vi "Write Default channels.vi"(8 "error in (no error)":errorcluster, 9 "Keep old\nplots":bool, 10 "Default channels":string[][](array[string]), 11 "Common Measurements in":refnum<class "Common Measurements.lvclass">) -> (0 "error out":errorcluster, 3 "Common Measurements out":refnum<class "Common Measurements.lvclass">)   [LabVIEW 2015, in "Common Measurements.lvclass"]
uses:
  Common Measurements.lvclass
  Common Measurements.lvclass/Common Measurements.ctl
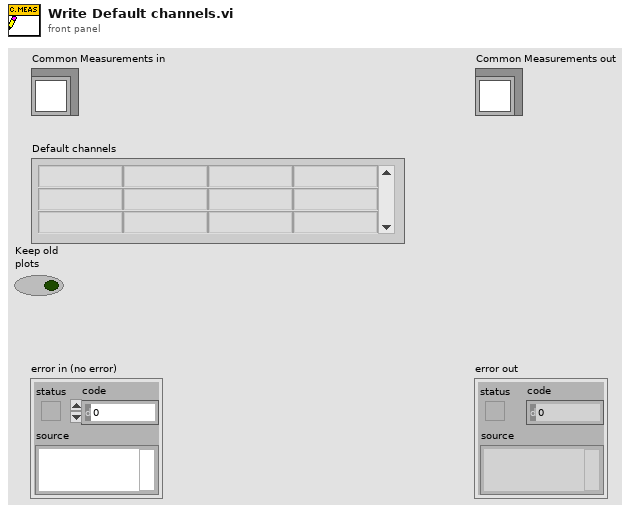
[diagram p1: front panel]
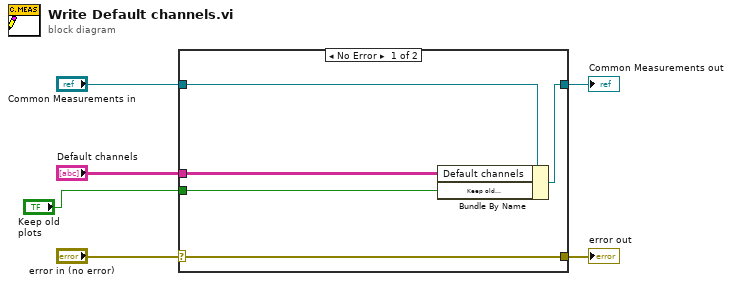
[diagram p0: block diagram]
diagram:
  n1 = case shown="No Error" "error in (no error)" {
    selector: "error in (no error)" -> [w11 w12]
    tunnel: [w11 w12] -> w5
    tunnel: [w9 w13] -> w3
    tunnel: "Common Measurements in" -> [w10 w13]
    tunnel: "Default channels" -> [w8 _]
    tunnel: "Keep old\nplots" -> [w7 _]
    frame No Error {
      n2 = Bundle By Name(cluster=w10, "Default channels"=w8, "Keep old\nplots"=w7) -> (w9:refnum<class "Common Measurements.lvclass">)
    }
    frame Error {
    }
  }
  "error out" <- w5
  "Common Measurements out" <- w3
